vi "TCP-IP Mgr.Send.vi"(8 "error in":errorcluster, 10 "Send Data":string, 11 "Q Name":string="TCP-IP Mgr") -> (0 "error out":errorcluster)   [LabVIEW 2024, in "EQMF.lvlib" / "TCP-IP.lvlib"]
uses:
  TCP-IP.lvlib
  Queues/Queue Utils.lvlib
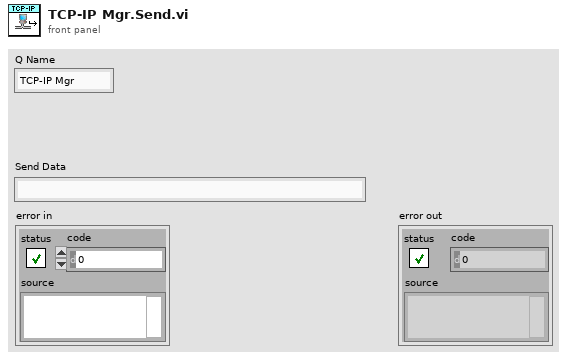
[diagram p1: front panel]
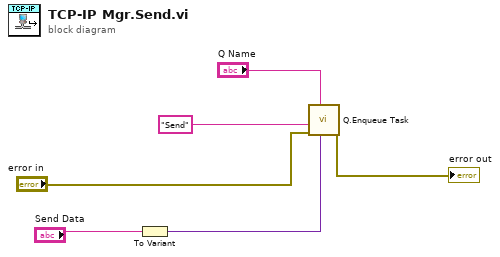
[diagram p0: block diagram]
diagram:
  n1 = To Variant(anything="Send Data") -> (Variant=w3:variant)
  n2 = call "Q.Enqueue Task.vi"("Data1"=w3, "Q Name"="Q Name", "Error In"="error in", "Task Name"="Send") -> ("error out"=→"error out":errorcluster)  [unwired: 6 in, 1 out]
